vi "Sensor DB xml.vi"() -> ()   [LabVIEW 2019]
uses:
  Common/DataTypes/Sensor LUT--cluster.ctl
  Common/DataTypes/Sensor database record--cluster.ctl
  Common/DataTypes/Sensor ranges--cluster.ctl
panel:
  in  "Sensor Records":T1=[{"name"="AEMC_1", "last updated"=timestamp(3690796694.047759 s since 1904-01-01), "manufacturer"="AEMC", "model"="MA-300-10-2-10 HF", "Sensitivity index"=1.0, "Sensor Ranges"={"Max.VOut.RMS (V)"=3.0, "Max.Out.Peak (V)"=4.246, "Sensitivity (mV/A)"=10.0, "Max.IOut.RMS(A)"=300.0, "Min.IOut.RMS(A)"=0.122}}, {"name"="AEMC_10", "last updated"=timestamp(3690796680 s since 1904-01-01), "manufacturer"="AEMC", "model"="MA-300-10-2-10 HF", "Sensitivity index"=10.0, "Sensor Ranges"={"Max.VOut.RMS (V)"=3.0, "Max.Out.Peak (V)"=4.246, "Sensitivity (mV/A)"=100.0, "Max.IOut.RMS(A)"=30.0, "Min.IOut.RMS(A)"=0.012}}, {"name"="PEM3_1", "last updated"=timestamp(3690796680 s since 1904-01-01), "manufacturer"="PEM", "model"="LFR03/3 B300", "Sensitivity index"=1.0, "Sensor Ranges"={"Max.VOut.RMS (V)"=6.0, "Max.Out.Peak (V)"=8.485, "Sensitivity (mV/A)"=10.0, "Max.IOut.RMS(A)"=600.0, "Min.IOut.RMS(A)"=0.122}}, {"name"="PEM3_10", "last updated"=timestamp(3690796680 s since 1904-01-01), "manufacturer"="PEM", "model"="LFR03/3 B300", "Sensitivity index"=10.0, "Sensor Ranges"={"Max.VOut.RMS (V)"=6.0, "Max.Out.Peak (V)"=8.485, "Sensitivity (mV/A)"=100.0, "Max.IOut.RMS(A)"=60.0, "Min.IOut.RMS(A)"=0.012}}, {"name"="PEM6_1", "last updated"=timestamp(3690796680 s since 1904-01-01), "manufacturer"="PEM", "model"="LFR06/6 B300", "Sensitivity index"=1.0, "Sensor Ranges"={"Max.VOut.RMS (V)"=6.0, "Max.Out.Peak (V)"=8.485, "Sensitivity (mV/A)"=5.0, "Max.IOut.RMS(A)"=1200.0, "Min.IOut.RMS(A)"=0.244}}, {"name"="PEM6_10", "last updated"=timestamp(3690796680 s since 1904-01-01), "manufacturer"="PEM", "model"="LFR06/6 B300", "Sensitivity index"=10.0, "Sensor Ranges"={"Max.VOut.RMS (V)"=6.0, "Max.Out.Peak (V)"=8.485, "Sensitivity (mV/A)"=50.0, "Max.IOut.RMS(A)"=120.0, "Min.IOut.RMS(A)"=0.024}}] {"last updated" format="%<%H:%M\n%d/%m/%Y>T"}
  in  "Config SettingsFile":path=path "C:/IHS_new/Config/Sensor XML Database.xml"
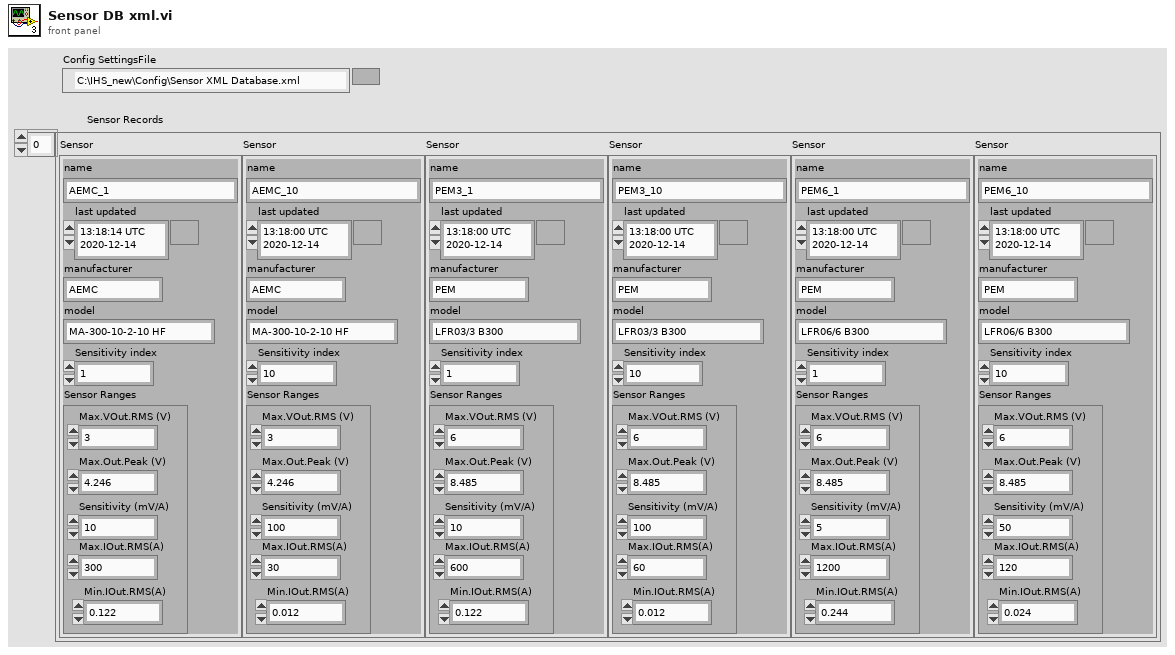
[diagram p1: front panel]
types:
  T1 = typedef "Sensor LUT--cluster.ctl" = T2[]
  T2 = typedef "Sensor database record--cluster.ctl" = cluster{"name":string, "last updated":timestamp, "manufacturer":string, "model":string, "Sensitivity index":dbl, "Sensor Ranges":T3}
  T3 = typedef "Sensor ranges--cluster.ctl" = cluster{"Max.VOut.RMS (V)":dbl, "Max.Out.Peak (V)":dbl, "Sensitivity (mV/A)":dbl, "Max.IOut.RMS(A)":dbl, "Min.IOut.RMS(A)":dbl}
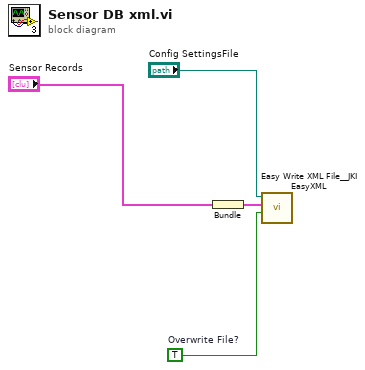
[diagram p0: block diagram]
diagram:
  w4 = TRUE  # Overwrite File?
  n1 = Bundle("Sensor Records"="Sensor Records") -> (w2:cluster{"Sensor Records":T1})  [unwired: 1 in]
  n2 = call <vilib>:"Easy Write XML File__JKI EasyXML.vi"("Overwrite File? (false)"=w4, "LabVIEW Data"=w2, "XML File Path"="Config SettingsFile") -> ()  [unwired: 7 in, 2 out]
